vi "verditempalert.vi"() -> ()   [LabVIEW 2013]
doc: "This VI alerts the user if the Verdi laser is overheating. The VI polls a voltage output from Barium that is +5V if the Verdi is overheating and 0V otherwise. Assuming the monitoring VI is running on Barium, this should alert the otherwise unsuspecting operator that the Verdi is having issues."
uses:
  <vilib>/DAQmx/read.llb/DAQmx Read (Analog DBL 1Chan 1Samp).vi
  <vilib>/DAQmx/miscellaneous.llb/DAQmx Fill In Error Info.vi
panel:
  out "Verdi Overheating?":bool
  out "+5 V indicates overheating.":dbl format="%0.2f"
  out "error out":errorcluster
  in  "error in":errorcluster
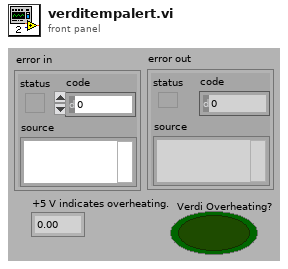
[diagram p1: front panel]
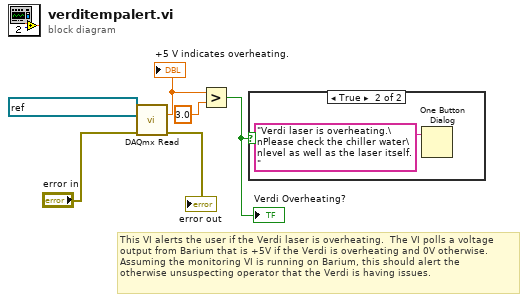
[diagram p0: block diagram]
diagram:
  # "This VI alerts the user if the Verdi laser is overheating.  The VI polls a voltage\noutput from Barium that is +5V if the Verdi is overheating and 0V otherwise.\nAssuming the monitoring VI is running on Barium, this should alert the\notherwise unsuspecting operator that the Verdi is having issues."
  n1 = call-poly <vilib>:"DAQmx Read.vi"("task/channels in"=refnum<k21> "VerdiTempMonitor", "error in"="error in") -> ("data"=w1:dbl, "error out"=→"error out":errorcluster)  [unwired: 11 in, 1 out]
  "+5 V indicates overheating." <- w1
  n2 = Greater?(x=w1, y=3.0 ("x")) -> (0:w3:bool)
  "Verdi Overheating?" <- w3
  n3 = case shown="True" w3 {
    frame False {
    }
    frame True {
      n4 = One Button Dialog(message="Verdi laser is overheating.\nPlease check the chiller water\nlevel as well as the laser itself.") -> ()  [unwired: 1 in, 1 out]
    }
  }
